vi "Create Configurable Actor.vi"(7 "Name":string, 8 "error in (no error)":errorcluster, 9 "Configuration":variant, 10 "ConfigManager":refnum<class "ConfigManager.lvclass">, 11 "ConfigurableActor":refnum<class "ConfigurableActor.lvclass">) -> (0 "error out":errorcluster, 3 "ConfigurableActor out":refnum<class "ConfigurableActor.lvclass">)   [LabVIEW 2014, in "ConfigurableActor.lvclass"]
uses:
  ConfigurableActor.lvclass
  <vilib>/LabVIEW Open Source/Configuration Manager/Manager/ConfigManager.lvclass
  ConfigurableActor.lvclass/ConfigurableActor.ctl
  <vilib>/LabVIEW Open Source Project/Unicity/UniqueName/UniqueNameClass/UniqueName.lvclass/UniqueName.ctl
  <vilib>/LabVIEW Open Source/Configuration Manager/Cache/ConfigManager.Cache.lvclass
  <vilib>/LabVIEW Open Source Project/Unicity/UniqueName/Registry/NameRegistry.lvclass
  <vilib>/LabVIEW Open Source Project/Unicity/UniqueName/UniqueNameClass/UniqueName.lvclass
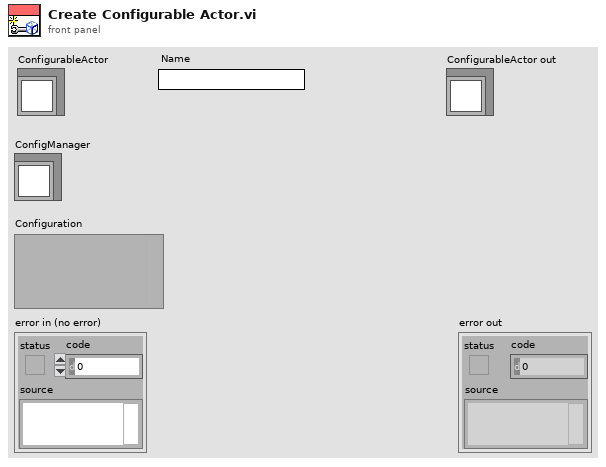
[diagram p1: front panel]
types:
  T1 = typedef "UniqueName.lvlib/NameRegistry.lvclass/RegistryConfiguration.ctl" = cluster{"Delimiter":refnum<class "Delimiter.lvclass">, "RandomStringGenerator":refnum<class "RandomStringGenerator.lvclass">, "UniquenessCriteria":refnum<class "UniquenessCriteria.lvclass">, "StringIncrement":refnum<class "StringIncrement.lvclass">}
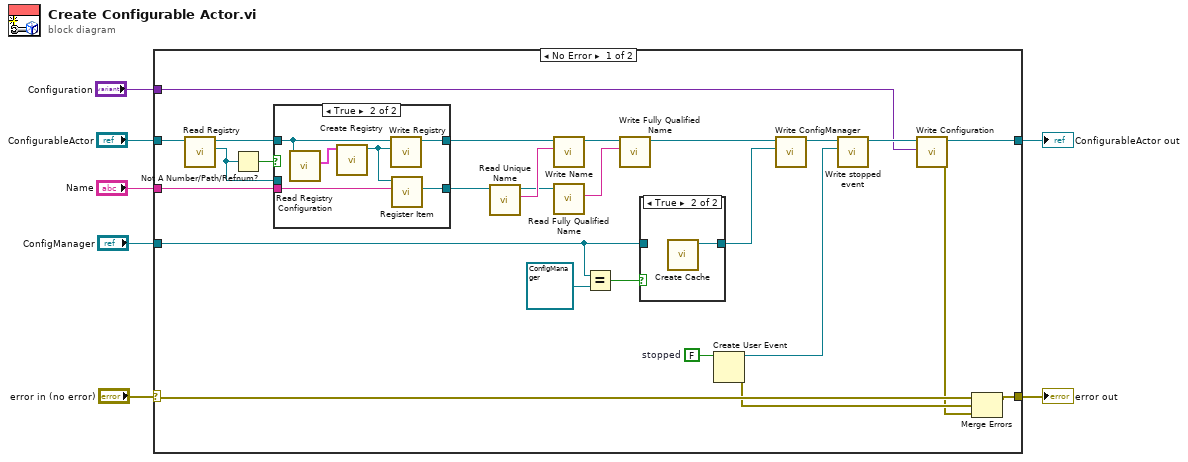
[diagram p0: block diagram]
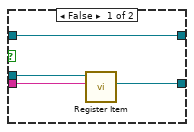
[diagram p2: hidden frame]
diagram:
  n1 = case shown="No Error" "error in (no error)" {
    selector: "error in (no error)" -> [w25 w46]
    tunnel: "ConfigurableActor" -> [w17 w47]
    tunnel: "ConfigManager" -> [w30 _]
    tunnel: [w20 w47] -> w5
    tunnel: [w26 w46] -> w3
    tunnel: "Name" -> [w9 _]
    tunnel: "Configuration" -> [w19 _]
    frame No Error {
      w29 = FALSE  # stopped
      n2 = call "Read Registry.vi"("ConfigurableActor in"=w17) -> ("Registry"=w13:refnum<data-value>, "ConfigurableActor out"=w16:refnum<class "ConfigurableActor.lvclass">)  [unwired: 9 in]
      n3 = Not A Number/Path/Refnum?(number/path/refnum=w13) -> (NaN/Path/Refnum?=w15:bool)
      n4 = case shown="True" w15 {
        tunnel: w16 -> [w37 w39]
        tunnel: [w37 w43] -> w14
        tunnel: w13 -> [w36 _]
        tunnel: w9 -> [w35 w40]
        tunnel: [w34 w41] -> w12
        frame False {
          n5 = call <vilib>:"Register Item.vi"("New Object Name"=w35, "Registry in"=w36) -> ("New Node"=w34:refnum<class "UniqueName.lvclass">)  [unwired: 7 in, 2 out]
        }
        frame True {
          n6 = call "Read Registry Configuration.vi"("ConfigurableActor in"=w39) -> ("Registry Configuration"=w38:T1)  [unwired: 9 in, 1 out]
          n7 = call <vilib>:"Create Registry.vi"("Registry Configuration"=w38) -> ("Registry"=w42:refnum<data-value>)  [unwired: 9 in, 1 out]
          n8 = call "Write Registry.vi"("Registry"=w42, "ConfigurableActor in"=w39) -> ("ConfigurableActor out"=w43:refnum<class "ConfigurableActor.lvclass">)  [unwired: 9 in]
          n9 = call <vilib>:"Register Item.vi"("New Object Name"=w40, "Registry in"=w42) -> ("New Node"=w41:refnum<class "UniqueName.lvclass">)  [unwired: 7 in, 2 out]
        }
      }
      n10 = call <vilib>:"Read Unique Name.vi"("UniqueName in"=w12) -> ("Unique Name"=w11:string, "UniqueName out"=w10:refnum<class "UniqueName.lvclass">)  [unwired: 9 in]
      n11 = call "Write Name.vi"("Name"=w11, "ConfigurableActor in"=w14) -> ("ConfigurableActor out"=w23:refnum<class "ConfigurableActor.lvclass">)  [unwired: 8 in, 1 out]
      n12 = call <vilib>:"Read Fully Qualified Name.vi"("UniqueName in"=w10) -> ("Fully Qualified Name"=w8:string)  [unwired: 9 in, 1 out]
      n13 = Equal?(x=w30, y=refnum<class "ConfigManager.lvclass"> refnum) -> (x = y?=w31:bool)
      n14 = call "Write Fully Qualified Name.vi"("Fully Qualified Name"=w8, "ConfigurableActor in"=w23) -> ("ConfigurableActor out"=w22:refnum<class "ConfigurableActor.lvclass">)  [unwired: 8 in, 1 out]
      n15 = case shown="True" w31 {
        tunnel: [w44 w45] -> w33
        tunnel: w30 -> [w44 _]
        frame False {
        }
        frame True {
          n16 = call <vilib>:"Create Cache.vi"() -> ("ConfigManager.Cache"=w45:refnum<class "ConfigManager.Cache.lvclass">)  [unwired: 11 in]
        }
      }
      n17 = Create User Event(user event datatype=w29) -> (user event=w27:refnum<user-event>, error out=w24:errorcluster)  [unwired: 1 in]
      n18 = call "Write ConfigManager.vi"("ConfigManager"=w33, "ConfigurableActor in"=w22) -> ("ConfigurableActor out"=w28:refnum<class "ConfigurableActor.lvclass">)  [unwired: 8 in, 1 out]
      n19 = call "Write stopped event.vi"("stopped event"=w27, "ConfigurableActor in"=w28) -> ("ConfigurableActor out"=w21:refnum<class "ConfigurableActor.lvclass">)  [unwired: 8 in, 1 out]
      n20 = call "Write Configuration.vi"("Type"=w19, "ConfigurableActor in"=w21) -> ("error out"=w18:errorcluster, "ConfigurableActor out"=w20:refnum<class "ConfigurableActor.lvclass">)  [unwired: 8 in]
      n21 = Merge Errors(w25, w24, w18) -> (w26:errorcluster)
    }
    frame Error {
    }
  }
  "ConfigurableActor out" <- w5
  "error out" <- w3
